vi "Build Text JSON for MCP.vi"(8 "error in (no error)":errorcluster, 11 "text in":string) -> (0 "error out":errorcluster, 3 "MCP JSON text content":string)   [LabVIEW 2025, in "MCP Server.lvlib"]
uses:
  MCP Server.lvlib
  <vilib>/JDP Science/JSONtext/JSONtext.lvlib
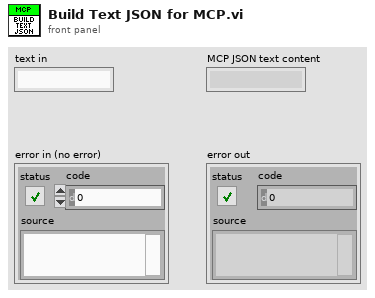
[diagram p1: front panel]
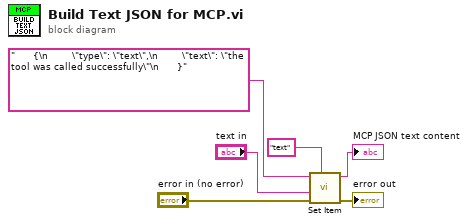
[diagram p0: block diagram]
diagram:
  n1 = call <vilib>:"Set Item.vi"("$Path or Item Name"="text", "error in (no error)"="error in (no error)", "JSON to Insert"="text in", "JSON"="      {\n        \"type\": \"text\",\n        \"text\": \"the tool was called successfully\"\n      }" ("element")) -> ("error out"=→"error out":errorcluster, "<JSON>"=→"MCP JSON text content":string)  [unwired: 4 in, 1 out]
